vi "Configure Device.vi"(8 "error in (no error)":errorcluster, 10 "Max beams":dbl, 11 "Device in":refnum<class "CK.lvclass">) -> (0 "error out":errorcluster, 3 "Device out":refnum<class "CK.lvclass">)   [LabVIEW 2020, in "CK.lvclass"]
doc: "Interface for configuring the device for testing"
uses:
  CK.lvclass
  Controls/Register to Write.ctl
  PIC-device/PIC-Device.lvclass
panel:
  in  "USID":bool=TRUE
  in  "label":string="Control for CK tuners" caption="text"
  out "Boolean array":bool[][](array[boolean])
  in  "Read Info":bool
  in  "OK Button":bool
  in  "Capa values":string="0:31/1" caption="Capacitance value (dec)"
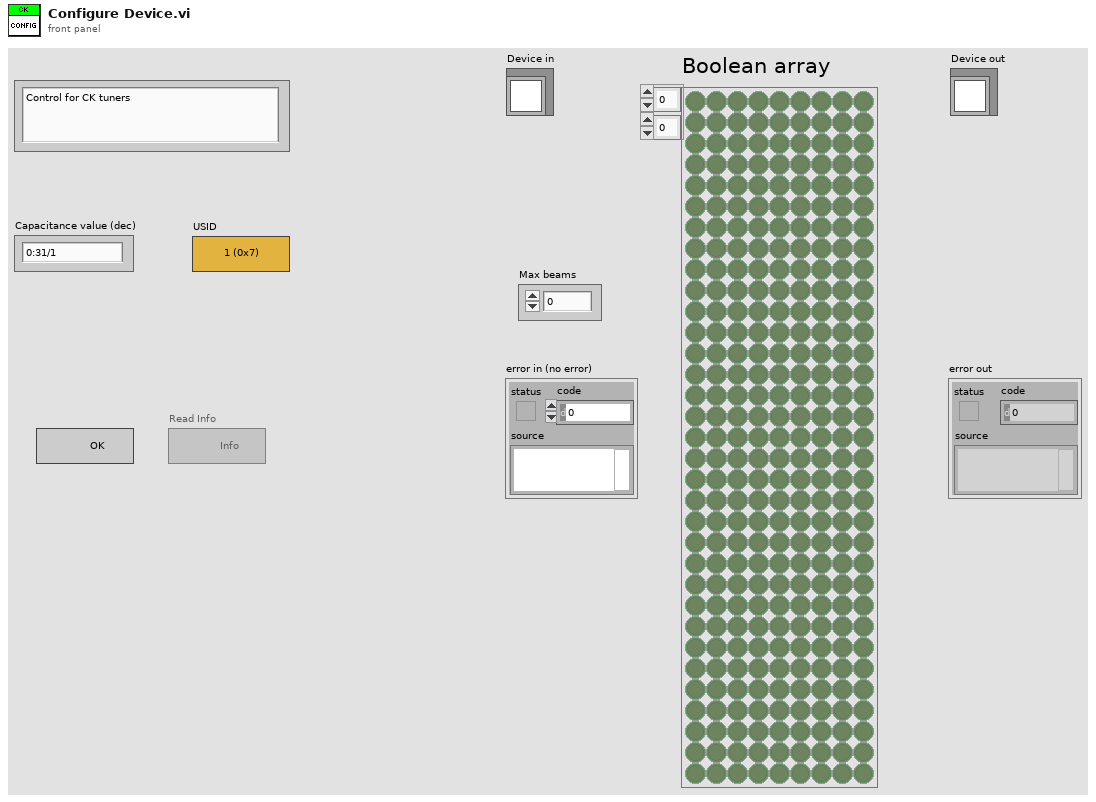
[diagram p1: front panel]
types:
  T1 = typedef "PIC-Device.lvclass/Register to Write.ctl" = cluster{"Register":u32, "Value":u32, "Dev Address":u32, "Physical Adress":u32}
  T2 = cluster{"Cap states reg":T1[], "Cap states":dbl[], "Cap sweep string":string}
  T3 = cluster{"Cap states reg":T1[], "Cap states":dbl[], "Cap sweep string":string}[]
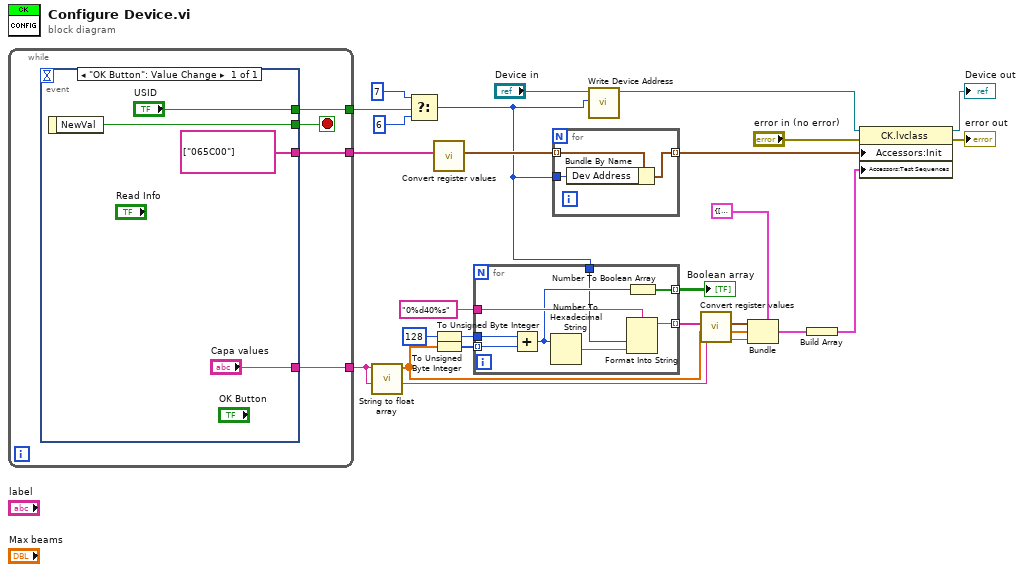
[diagram p0: block diagram]
diagram:
  n1 = while {
    tunnel: [w27] -> w16
    tunnel: [w26] -> w12
    tunnel: [w25] -> w4
    stop <- w28 stop-if-true
    n2 = event shown="[0] \"OK Button\": Value Change" {
      selector: _ -> [_]
      dyn-events: _ -> [_]
      timeout: _ -> [_]
      tunnel: [w32] -> w28
      tunnel: [string[] ["065C00"] ("Opening sequence")] -> w27
      tunnel: ["Capa values"] -> w26
      tunnel: ["USID"] -> w25
      event "OK Button": Value Change {
        n3 = event-data() -> ("NewVal"=w32:bool)  [unwired: 1 in]
      }
    }
  }
  n4 = call "String to float array.vi"("String"=w12) -> ("Array - Numeric"=w24:dbl[])  [unwired: 9 in, 1 out]
  n5 = Select(t=u8 7 ("Device Address"), s=w4, f=u8 6 ("Device Address")) -> (s? t:f=w2:u8)
  n6 = call "Convert register values.vi"("Register strings"=w16) -> ("Register clusters out"=w3:T1[])  [unwired: 9 in, 1 out]
  n7 = To Unsigned Byte Integer(number=u8 128) -> (unsigned 8bit integer=w19:u8)
  n8 = To Unsigned Byte Integer(number=w24) -> (unsigned 8bit integer=w18:u8[])
  n9 = for {
    tunnel: w18 -> [w36] mode=indexing
    tunnel: "0%d40%s" -> [w40]
    tunnel: [w39] -> w20 mode=indexing
    tunnel: w19 -> [w38]
    tunnel: [w34] -> w22 mode=indexing
    tunnel: w2 -> [w33]
    n10 = Add(x=w38, y=w36) -> (x+y=w37:u8)
    n11 = Number To Hexadecimal String(2:w37) -> (0:w35:string)  [unwired: 1 in]
    n12 = Format Into String(format string=w40, w33, w35) -> (resulting string=w34:string)  [unwired: 2 in, 1 out]
    n13 = Number To Boolean Array(number=w37) -> (Boolean array=w39:bool[])
  }
  "Boolean array" <- w20
  n14 = for {
    tunnel: w3 -> [w43] mode=indexing
    tunnel: w2 -> [w42]
    tunnel: [w41] -> w1 mode=indexing
    n15 = Bundle By Name(cluster=w43, "Dev Address"=w42) -> (w41:T1)
  }
  n16 = call-dynamic "Write Device Address.vi"("Device Address"=w2, "PIC-Device in"="Device in") -> ("PIC-Device out"=w7:refnum<class "CK.lvclass">)  [unwired: 9 in]
  n17 = call "Convert register values.vi"("Register strings"=w22) -> ("Register clusters out"=w23:T1[])  [unwired: 9 in, 1 out]
  n18 = Bundle(cluster=T2 {"Cap states reg"=[{"Register"=0, "Value"=0, "Dev Address"=7, "Physical Adress"=0}, {"Register"=0, "Value"=128, "Dev Address"=7, "Physical Adress"=0}], "Cap states"=[], "Cap sweep string"=""} ("Test Sequence"), "Cap states reg"=w23, "Cap states"=w24, "Cap sweep string"=w12) -> (w21:T2)
  n19 = Build Array(w21) -> (w17:T3)
  n20 = property class="CK.lvclass"(reference=w7, error in="error in (no error)", "Accessors:Init"=w1, "Accessors:Test Sequences"=w17) -> (reference out=→"Device out":refnum<class "CK.lvclass">, error out=→"error out":errorcluster)
